vi "PID Gain Schedule (DBL).vi"(4 "PID gain schedule":T1(array[cluster])=[{"PID gains"={"proportional gain (Kc)"=1.0, "integral time (Ti, min)"=0.01, "derivative time (Td, min)"=0.0}, "max value"=100.0}] {"max value" format="%.2f"; "PID gains"."derivative time (Td, min)" format="%.3f"; "PID gains"."integral time (Ti, min)" format="%.3f"; "PID gains"."proportional gain (Kc)" format="%.3f"}, 5 "gain scheduling value":dbl format="%.2f") -> (1 "PID gains out":T2={"proportional gain (Kc)"=1.0, "integral time (Ti, min)"=0.01, "derivative time (Td, min)"=0.0} {"derivative time (Td, min)" format="%.3f"; "integral time (Ti, min)" format="%.3f"; "proportional gain (Kc)" format="%.3f"}, 2 "index out":i32)   [LabVIEW 2020, in "NI_PID_pid.lvlib"]
doc: "Selects a set of PID gains from a gain schedule for the control of processes that require different sets of gains for different regions of operation, such as highly nonlinear processes. Use the DBL instance of this VI to implement a single control loop. Use the DBL Array instance to implement parallel multi-loop control."
uses:
  NI_PID_pid.lvlib
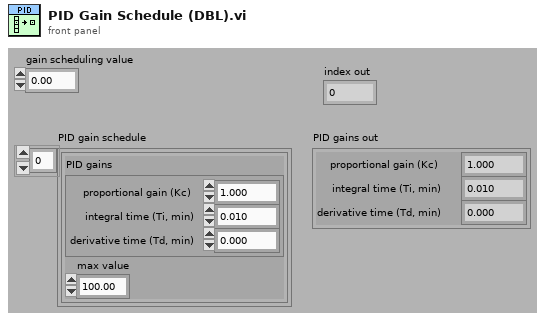
[diagram p1: front panel]
types:
  T1 = cluster{"PID gains":cluster{"proportional gain (Kc)":dbl, "integral time (Ti, min)":dbl, "derivative time (Td, min)":dbl}, "max value":dbl}[]
  T2 = cluster{"proportional gain (Kc)":dbl, "integral time (Ti, min)":dbl, "derivative time (Td, min)":dbl}
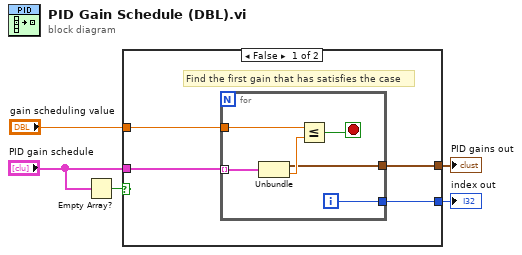
[diagram p0: block diagram]
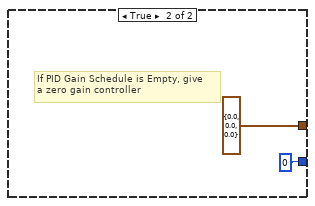
[diagram p2: hidden frame]
diagram:
  n1 = Empty Array?(array="PID gain schedule") -> (empty?=w2:bool)
  n2 = case shown="False" w2 {
    tunnel: "gain scheduling value" -> [w9 _]
    tunnel: [w8 T2 {"proportional gain (Kc)"=0.0, "integral time (Ti, min)"=0.0, "derivative time (Td, min)"=0.0} ("PID gains")] -> w4
    tunnel: "PID gain schedule" -> [w7 _]
    tunnel: [w6 0] -> w1
    frame False {
      # "Find the first gain that has satisfies the case"
      n3 = for {
        tunnel: w7 -> [w15] mode=indexing
        tunnel: w9 -> [w14]
        tunnel: [w12] -> w8
        tunnel: [w11] -> w6
        i -> [w11]
        stop <- w10 stop-if-true
        n4 = Unbundle(w15) -> ("PID gains"=w12:T2, "max value"=w13:dbl)
        n5 = Less Or Equal?(x=w14, y=w13) -> (x <= y?=w10:bool)
      }
    }
    frame True {
      # "If PID Gain Schedule is Empty, give\na zero gain controller"
    }
  }
  "PID gains out" <- w4
  "index out" <- w1
